vi "fgv_gps_receive-arr_buff.vi"(7 "cmd":enum16{"read", "write utm", "write heading"}(ring), 11 "gps receive str":string) -> (2 "protocol arrary":string[](array[string]), 3 "gps log out":string)   [LabVIEW 2019]
panel:
  out "str arr":string[](array[string])=["USB3", "0", "47.0", "FINESTEERING", "2113", "382087.450", "02000000", "471d", "15824;INS_SOLUTION_GOOD", "INS_RTKFIXED", "37.37018090370", "126.72087216668", "9.8880", "22.3000", "0.0830", "0.0260", "-0.0115", "-0.214462895", "-0.641533972", "40.858445824", "0.1537", "0.1609", "0.1285", "0.0368", "0.0362", "0.0228", "0.0337", "0.0332", "0.1017", "0f000041", "0*1332c6d8"]
  out "GNSS time":string="382087.450"
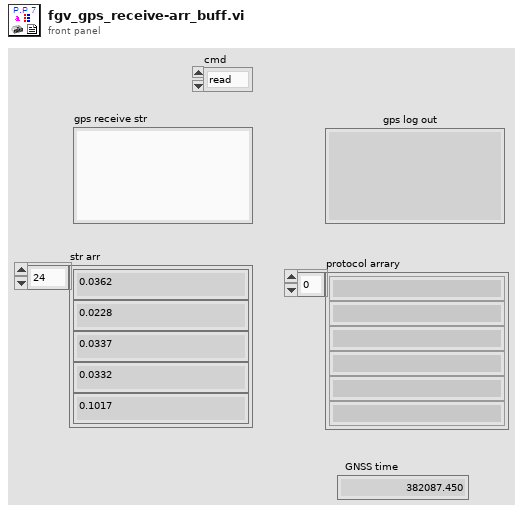
[diagram p1: front panel]
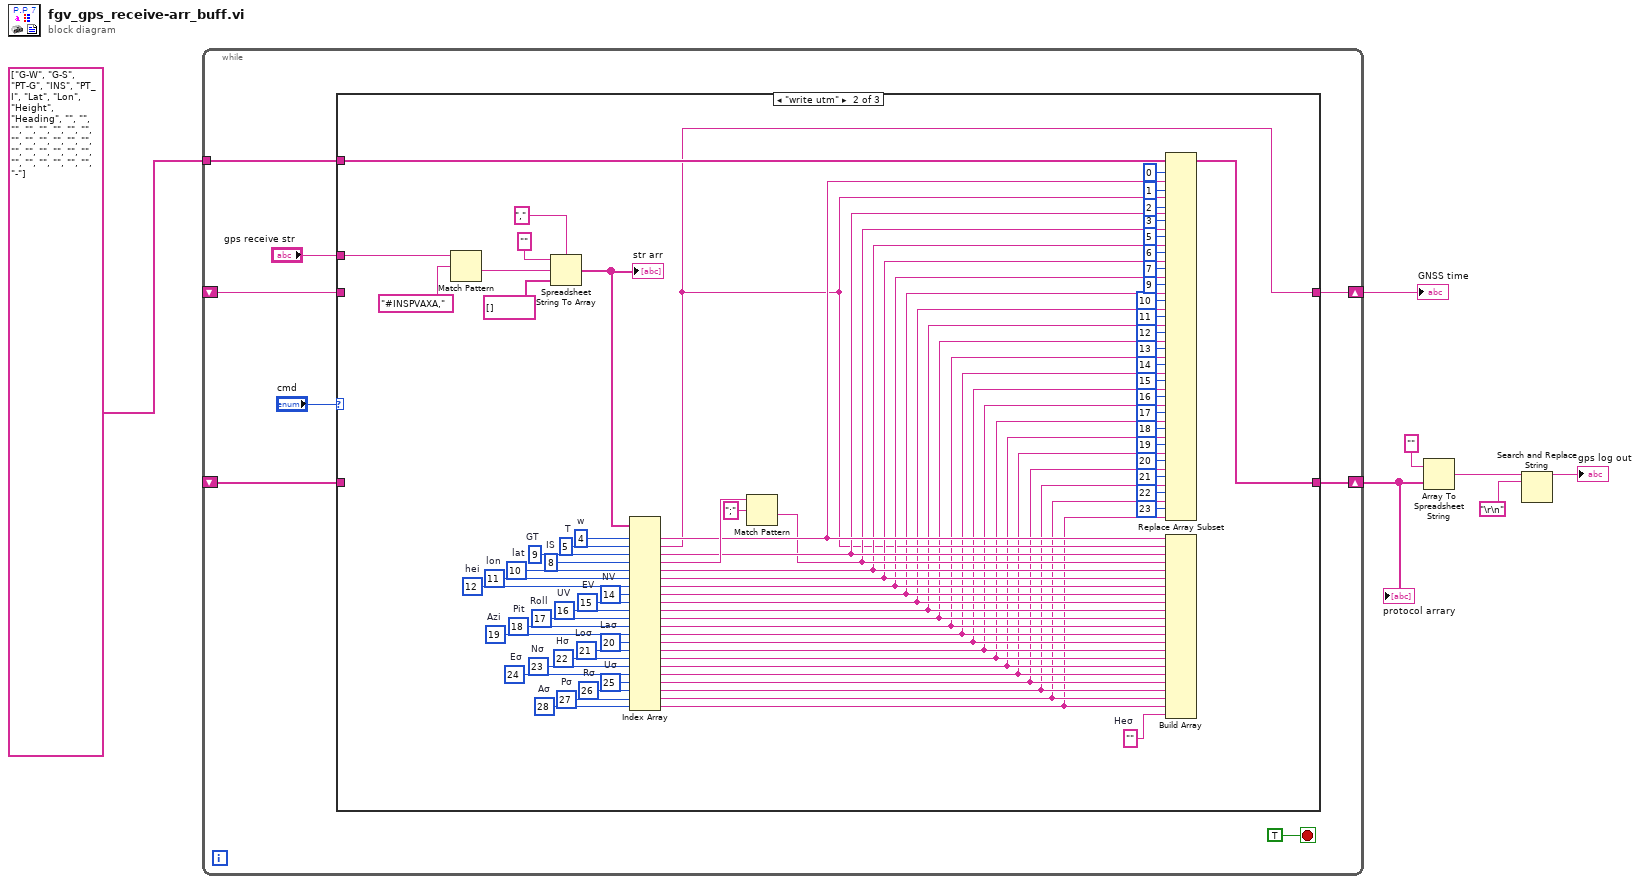
[diagram p0: block diagram]
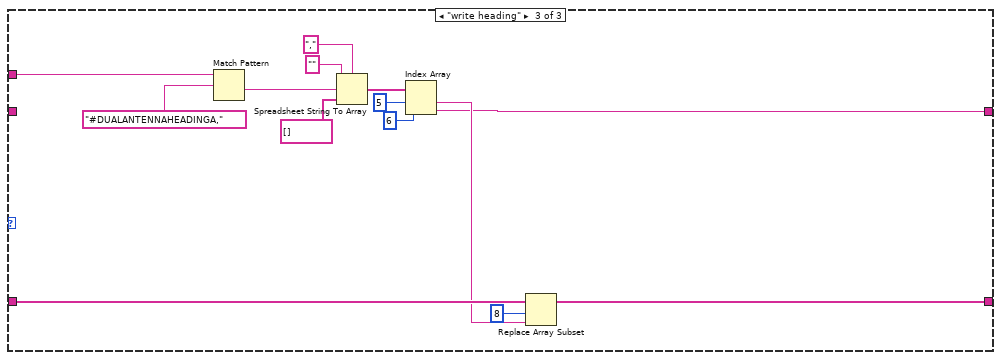
[diagram p3: hidden frame]
diagram:
  n1 = while {
    shift-right: [w14] -> w2
    shift-left: _ -> [w13]
    shift-right: [w11] -> w7
    shift-left: _ -> [w10]
    tunnel: string[] ["G-W", "G-S", "PT-G", "INS", "PT_I", "Lat", "Lon", "Height", "Heading", "", "", "", "", "", "", "", "", "", "", "", "", "", "", "", "", "", "", "", "", "", "", "", "", "", "", "-"] -> [w8]
    stop <- TRUE stop-if-true
    n2 = case shown="\"write utm\"" "cmd" {
      tunnel: [w17 w63 w103] -> w14
      tunnel: w13 -> [w17 _ w104]
      tunnel: [w16 w48 w96] -> w11
      tunnel: w10 -> [w16 _ _]
      tunnel: "gps receive str" -> [_ w64 w98]
      tunnel: w8 -> [_ w62 _]
      frame "read", Default {
      }
      frame "write utm" {
        w65 = ""  # Heσ
        w66 = 28  # Aσ
        w67 = 27  # Pσ
        w68 = 26  # Rσ
        w69 = 25  # Uσ
        w70 = 24  # Eσ
        w71 = 23  # Nσ
        w72 = 22  # Hσ
        w73 = 21  # Loσ
        w74 = 20  # Laσ
        w75 = 19  # Azi
        w76 = 18  # Pit
        w77 = 17  # Roll
        w78 = 16  # UV
        w79 = 15  # EV
        w80 = 14  # NV
        w81 = 12  # hei
        w82 = 11  # lon
        w83 = 10  # lat
        w86 = 8  # IS
        w87 = 9  # GT
        w88 = 5  # T
        w89 = 4  # w
        n3 = Match Pattern(string=w64, regular expression="#INSPVAXA," ("정규식")) -> (after substring=w94:string)  [unwired: 1 in, 3 out]
        n4 = Spreadsheet String To Array(delimiter (Tab)="," ("구분 문자 (탭)"), format string="" ("포맷 문자열"), spreadsheet string=w94, array type (2D Dbl)=string[] []) -> (array=w90:string[])
        "str arr" <- w90
        n5 = Index Array(array=w90, index #1=w89, index #2=w88, index #3=w87, index #4=w86, index #5=w83, index #6=w82, index #7=w81, index #8=w80, index #9=w79, index #10=w78, index #11=w77, index #12=w76, index #13=w75, index #14=w74, index #15=w73, index #16=w72, index #17=w71, index #18=w70, index #19=w69, index #20=w68, index #21=w67, index #22=w66) -> (element #1=w61:string, element #2=w48:string, element #3=w60:string, element #4=w85:string, element #5=w56:string, element #6=w55:string, element #7=w49:string, element #8=w46:string, element #9=w44:string, element #10=w37:string, element #11=w36:string, element #12=w35:string, element #13=w34:string, element #14=w33:string, element #15=w32:string, element #16=w28:string, element #17=w27:string, element #18=w26:string, element #19=w24:string, element #20=w22:string, element #21=w20:string, element #22=w18:string)
        n6 = Match Pattern(string=w85, regular expression=";" ("정규식")) -> (after substring=w59:string)  [unwired: 1 in, 3 out]
        n7 = Replace Array Subset(array=w62, new element #1=w61, index #1=0 ("인덱스"), new element #2=w48, index #2=1 ("인덱스"), new element #3=w60, index #3=2 ("인덱스"), new element #4=w59, index #4=3 ("인덱스"), new element #5=w56, index #5=5 ("인덱스"), new element #6=w55, index #6=6 ("인덱스"), new element #7=w49, index #7=7 ("인덱스"), new element #8=w46, index #8=9 ("인덱스"), new element #9=w44, index #9=10 ("인덱스"), new element #10=w37, index #10=11 ("인덱스"), new element #11=w36, index #11=12 ("인덱스"), new element #12=w35, index #12=13 ("인덱스"), new element #13=w34, index #13=14 ("인덱스"), new element #14=w33, index #14=15 ("인덱스"), new element #15=w32, index #15=16 ("인덱스"), new element #16=w28, index #16=17 ("인덱스"), new element #17=w27, index #17=18 ("인덱스"), new element #18=w26, index #18=19 ("인덱스"), new element #19=w24, index #19=20 ("인덱스"), new element #20=w22, index #20=21 ("인덱스"), new element #21=w20, index #21=22 ("인덱스"), new element #22=w18, index #22=23 ("인덱스")) -> (w63:string[])
        n8 = Build Array(w61, w48, w60, w59, w56, w55, w49, w46, w44, w37, w36, w35, w34, w33, w32, w28, w27, w26, w24, w22, w20, w18, w65) -> ()  [unwired: 1 out]
      }
      frame "write heading" {
        n9 = Match Pattern(string=w98, regular expression="#DUALANTENNAHEADINGA," ("정규식")) -> (after substring=w109:string)  [unwired: 1 in, 3 out]
        n10 = Spreadsheet String To Array(delimiter (Tab)="," ("구분 문자 (탭)"), format string="" ("포맷 문자열"), spreadsheet string=w109, array type (2D Dbl)=string[] []) -> (array=w101:string[])
        n11 = Index Array(array=w101, index #1=5 ("인덱스"), index #2=6 ("인덱스")) -> (element #1=w99:string, element #2=w96:string)
        n12 = Replace Array Subset(array=w104, new element=w99, index=8 ("인덱스")) -> (w103:string[])
      }
    }
  }
  "GNSS time" <- w7
  "protocol arrary" <- w2
  n13 = Array To Spreadsheet String(array=w2, 3:"" ("포맷 문자열")) -> (spreadsheet string=w5:string)  [unwired: 1 in]
  n14 = Search and Replace String(input string=w5, search string="\r\n") -> (result string=→"gps log out":string)  [unwired: 6 in, 3 out]
